vi "set_motors.vi"(8 "error in (no error)":errorcluster, 9 "SHG":i32=201790, 10 "resonator":i32=927080) -> (0 "error out":errorcluster, 2 "fundamental (nm)":dbl=536.684118137483 format="%.4f")   [LabVIEW 2017, in "sirah.lvlib"]
uses:
  Sirah_Control_26/Sirah Control Classic 2.6/LabVIEW/Laser/Laser Library LabVIEW 7.1/Stage Reference.ctl
  Sirah_Control_26/Sirah Control Classic 2.6/LabVIEW/Laser/Laser Library LabVIEW 7.1/Laser Position Mode.ctl
  sirah.lvlib
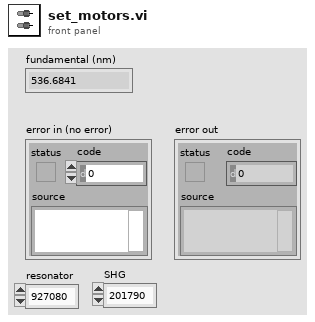
[diagram p1: front panel]
types:
  T1 = enum16{"absolute", "relative", "absolute, quick", "relative, quick"}
  T2 = typedef "Stage Reference.ctl" = enum16{"Resonator", "Conversion(1)", "Conversion(2)", "Conversion(3)", "Conversion(4)", "Conversion(5)", "Conversion(6)", "Conversion(7)"}
  T3 = typedef "Laser Position Mode.ctl" = enum16{"fundamental, wavelength / nm", "fundamental, wavenumber / cm-1", "fundamental, frequency / GHz", "SHG, wavelength / nm", "SHG, wavenumber /  cm-1", "SHG, frequency / GHz", "DFM @ 1064 nm, wavelength / nm", "DFM @ 1064 nm, wavenumber / cm-1", "DFM @ 1064 nm, freuency / GHz", "OPA @ 1064 nm, wavelength / nm", "OPA @ 1064 nm, wavenumber / cm-1", "OPA @ 1064 nm, frequency / GHz", "THG, wavelength / nm", "THG, wavenumber / cm-1", "THG, frequency / GHz", "SFM @ 1064 nm, wavelength / nm", "SFM @ 1064 nm, wavenumber / cm-1", "SFM @ 1064 nm, frequency / GHz", "SFM @ 532 nm, wavelength / nm", "SFM @ 532 nm, wavenumber / cm-1", "SFM @ 532 nm, frequency / GHz", "SFM @ 355 nm, wavelength / nm", "SFM @ 355 nm, wavenumber / cm-1", "SFM @ 355 nm, frequency / GHz", "SFM @ 266 nm, wavelength / nm", "SFM @ 266 nm, wavenumber / cm-1", "SFM @ 266 nm, frequency / GHz", "NIR, wavelength / nm", "NIR, wavenumber / cm-1", "NIR, frequency / GHz", "DFM @ 355 nm, wavelength / nm", "DFM @ 355 nm, wavenumber / cm-1", "DFM @ 355 nm, frequency / GHz", "MAD @ 1064 nm, wavelength / nm", "MAD @ 1064 nm, wavenumber / cm-1", "MAD @ 1064 nm, frequency / GHz"}
  T4 = typedef "Laser Reference.ctl" = refnum<k4>
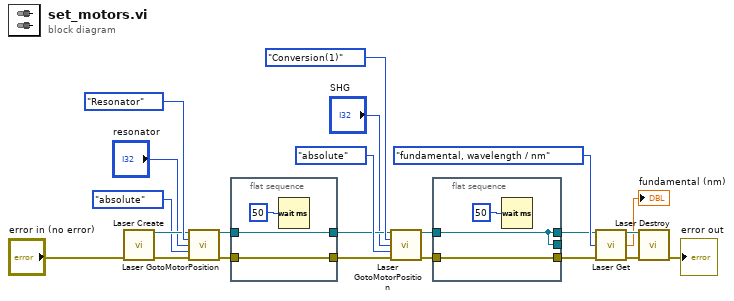
[diagram p0: block diagram]
diagram:
  n1 = call "Laser Create.vi"("error in (no error)"="error in (no error)") -> ("laser out"=w16:T4, "error out"=w14:errorcluster)  [unwired: 13 in]
  n2 = call "Laser GotoMotorPosition.vi"("laser"=w16, "stage ID"=Stage_Reference."Resonator", "position"="resonator", "mode"=T1."absolute", "error in (no error)"=w14) -> ("laser out"=w11:T4, "error out"=w12:errorcluster)  [unwired: 9 in]
  n3 = flat-sequence {
    tunnel: [w25] -> w6
    tunnel: w12 -> [w25]
    tunnel: w11 -> [w24]
    tunnel: [w24] -> w7
    frame #0 {
      n4 = Wait (ms)(milliseconds to wait=u32 50) -> ()  [unwired: 1 out]
    }
  }
  n5 = call "Laser GotoMotorPosition.vi"("laser"=w7, "stage ID"=Stage_Reference."Conversion(1)", "position"="SHG", "mode"=T1."absolute", "error in (no error)"=w6) -> ("laser out"=w4:T4, "error out"=w5:errorcluster)  [unwired: 9 in]
  n6 = flat-sequence {
    tunnel: [w28] -> w2
    tunnel: w5 -> [w28]
    tunnel: w4 -> [w26]
    tunnel: [w26] -> _
    tunnel: [w26] -> w3
    frame #0 {
      n7 = Wait (ms)(milliseconds to wait=u32 50) -> ()  [unwired: 1 out]
    }
  }
  n8 = call "Laser Get.vi"("laser"=w3, "laser position mode (fundamental wavelength)"=Laser_Position_Mode."fundamental, wavelength / nm", "error in (no error)"=w2) -> ("laser out"=w22:T4, "position"=→"fundamental (nm)":dbl, "error out"=w20:errorcluster)  [unwired: 10 in]
  n9 = call "Laser Destroy.vi"("laser"=w22, "error in (no error)"=w20) -> ("error out"=→"error out":errorcluster)  [unwired: 13 in]
